vi "Sys B RX Host.vi"() -> ()   [LabVIEW 2019]
uses:
  SubVIs/mmWave HW Control/HW RX resources cluster.ctl
  <instrlib>/niMmWave/ni3610 and ni3630/controls/public/Board Information.ctl
  <instrlib>/niMmWave/ni3610 and ni3630/private/mm/Typedefs/PID.ctl
  <instrlib>/niMmWave/ni3610 and ni3630/controls/private/Board Hardware Revision.ctl
  SubVIs/mmWave HW Control/HW RX RF config cluster.ctl
  SubVIs/mmWave HW Control/HW Timing module config cluster.ctl
  SubVIs/mmWave HW Control/RX acquisition config.ctl
  SubVIs/Low-level/TypeDefs/TX trigger config.ctl
  FPGA/SubVIs/Utility/FPGA driver trigger source.ctl
  FPGA/SubVIs/Utility/FPGA driver trigger destination.ctl
  SubVIs/mmWave HW Control/Message and Data cluster.ctl
  SubVIs/mmWave HW Control/HW state enum.ctl
  <vilib>/Utility/error.llb/DialogType.ctl
  SubVIs/Low-level/TypeDefs/Hardware Configuration.ctl
  SubVIs/Low-level/TypeDefs/Direction.ctl
  SubVIs/Low-level/TypeDefs/Resources.ctl
  <vilib>/userdefined/High Color/nirio_resource_hc.ctl
  SubVIs/Low-level/TypeDefs/Front End Configuration.ctl
  SubVIs/Low-level/TypeDefs/Channel Configuration.ctl
  <instrlib>/niMmWave/ni3620/Config/v1/Host/Public/Typedefs/mmWave Port.ctl
  Intertarget communication/NS slave_class/NS slave.lvclass
  C:/Barkhausen mmWave radar/Development/LV/Barkhausen mmWave hardware control/Host/Intertarget communication/CR slave_class/CR slave.lvclass
  SubVIs/mmWave HW Control/mmWave HW Control.lvlib
  <instrlib>/niMmWave/ni3610 and ni3630/ni3610_and_ni3630_Driver_Lib.lvlib
  <instrlib>/niMmWave/ni3620/Config/v1/Host/niMmWave Config v1 Host.lvlib
  FPGA/SubVIs/Utility/FPGA Utility.lvlib
panel:
  out "SysA connected":bool
  in  "RX.Stop":bool
  out "Elements Remaining":u32
  out "Samples":u32
  in  "Stop Button":bool
  out "error out":T1
  out "Waveform plot":sgl[][](graph)
  in  "Tab Control":enum32{"HW setup", "Trigger setup"}(tab)
  in  "HW.RX resources":T2={"HW.IF"="IF_mod", "HW.ADC"="Rx_ADC", "HW.RX FPGA"="RX_FPGA"} caption="Reciever resources"
  in  "RX config":T3={"Gain"=0.0, "Frequency"=76000000000.0, "mmWave adapter"="mmWave0/0"} {"Frequency" format="%#_6fdb"; "Gain" format="%#_gdb"}
  in  "HW.init":bool
  in  "hw.conf trig":bool
  in  "HW.trig share config":T4={"mode"=enum."Import trig", "Timing module"="Dev1", "PXI line"="PXI_Trig1", "Module terminal"="PFI2"}
  in  "RX trigger options":T5={"delay"=136.0, "trig source"=enum."PXI_Trig", "PXI src"=1, "export"=enum."None", "PXI dest"=0}
  in  "Plot":bool=TRUE
  out "dt":dbl format="%#_6ps"
  in  "RX.read config":T8={"Samples"=16000}
  in  "RX.start":bool
  out "Rx information":T9={"product code"=30639, "hardware revision"=enum."Unknown", "serial number"=""} {"product code" items=["PXIe-3610 I/Q Generator"=30638, "PXIe-3630 I/Q Digitizer"=30639]}
  out "State":string
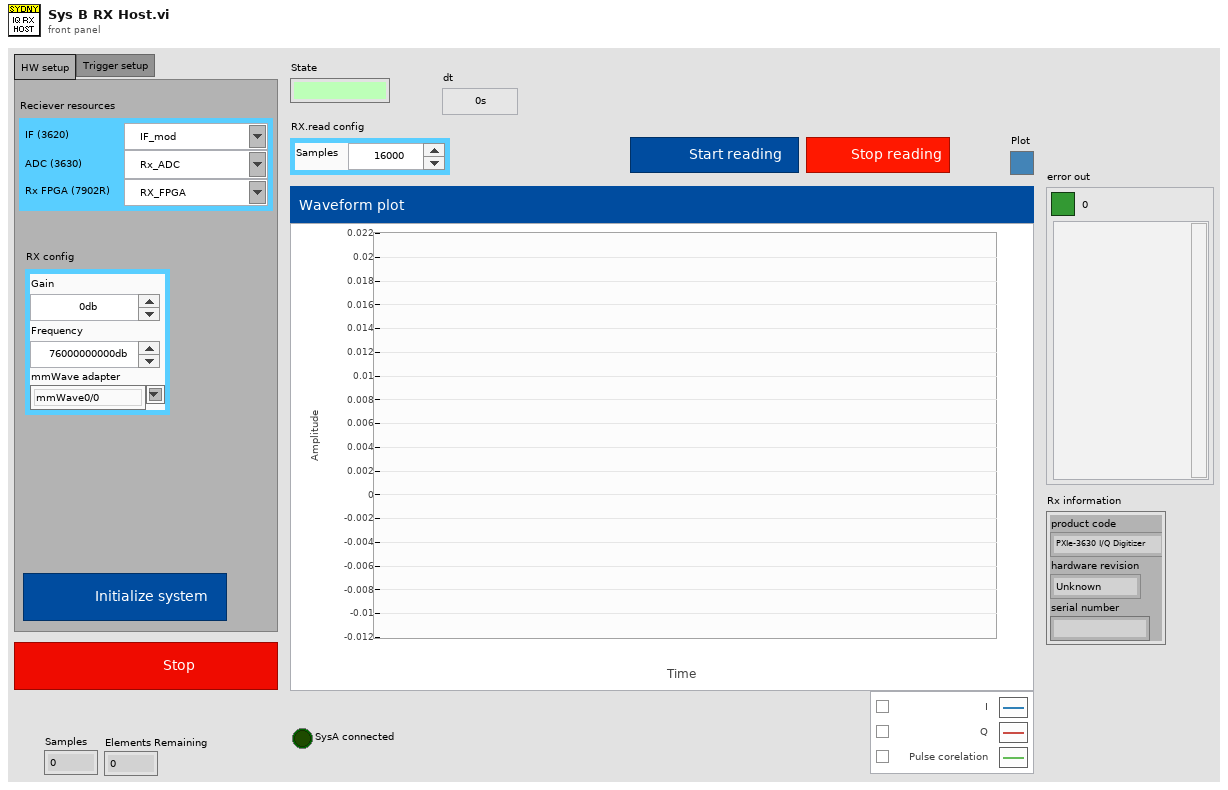
[diagram p1: front panel]
types:
  T1 = cluster{"Boolean Round":bool, "code":i32, "source":string}
  T2 = typedef "mmWave HW Control.lvlib/HW RX resources cluster.ctl" = cluster{"HW.IF":tag, "HW.ADC":refnum<visa-resource-name>, "HW.RX FPGA":tag}
  T3 = typedef "mmWave HW Control.lvlib/HW RX RF config cluster.ctl" = cluster{"Gain":dbl, "Frequency":dbl, "mmWave adapter":string}
  T4 = typedef "mmWave HW Control.lvlib/HW Timing module config cluster.ctl" = cluster{"mode":enum16{"None", "Export trig", "Import trig"}, "Timing module":tag, "PXI line":string, "Module terminal":string}
  T5 = typedef "TX trigger config.ctl" = cluster{"delay":dbl, "trig source":T6, "PXI src":i32, "export":T7, "PXI dest":i32}
  T6 = typedef "FPGA Utility.lvlib/FPGA driver trigger source.ctl" = enum16{"Use Tclk", "PXI_Trig", "Aurora RX trig"}
  T7 = typedef "FPGA Utility.lvlib/FPGA driver trigger destination.ctl" = enum16{"None", "Source trig", "Synced trig", "Delayed sync"}
  T8 = typedef "mmWave HW Control.lvlib/RX acquisition config.ctl" = cluster{"Samples":u32}
  T9 = typedef "Board Information.ctl" = cluster{"product code":T10, "hardware revision":T11, "serial number":string}
  T10 = typedef "ni3610_and_ni3630_Driver_Lib.lvlib/PID.ctl" = u16
  T11 = typedef "Board Hardware Revision.ctl" = enum16{"Unknown", "A", "B", "C", "D", "E", "F", "G", "H"}
  T12 = typedef "mmWave HW Control.lvlib/Message and Data cluster.ctl" = cluster{"message":string, "data":variant}
  T13 = typedef "mmWave HW Control.lvlib/HW state enum.ctl" = enum16{"idle", "configuration", "running", "exit"}
  T14 = typedef "Resources.ctl" = cluster{"7902R (Tx)":T15, "3610 (Tx)":refnum<visa-resource-name>, "3620 (IF)":T15, "3630 (RX)":refnum<visa-resource-name>, "7902R (Rx)":T15}
  T15 = typedef "nirio_resource_hc.ctl" = tag
  T16 = typedef "niMmWave Config v1 Host.lvlib/mmWave Port.ctl" = string
  T17 = typedef "Front End Configuration.ctl" = cluster{"port select":enum16{"IF Port", "Loopback", "Sync Port"}, "Rx hardware configuration":T18, "Tx hardware configuration":T18}
  T18 = typedef "Channel Configuration.ctl" = cluster{"gain (dB)":dbl, "frequency (Hz)":dbl, "mmWave adapter":string, "adapter active port":T16}
  T19 = typedef "DialogType.ctl" = u16
  T20 = typedef "Hardware Configuration.ctl" = cluster{"direction":T21, "baseband only":bool}
  T21 = typedef "Direction.ctl" = enum16{"Transceiver", "Receiver", "Transmitter"}
  T22 = typedef "Session.ctl" = cluster{"3620 session":refnum<queue>, "tx baseband session":T23, "rx baseband session":T31, "tx gain (dB)":dbl, "rx gain (dB)":dbl, "hardware configuration":T20, "gain ranging":T32[], "pxi trigger bus information":T33}
  T23 = typedef "Tx Baseband Session.ctl" = cluster{"3610 session":T24, "7902 reference":T30}
  T24 = typedef "ni3610_and_ni3630_Driver_Lib.lvlib/Main Settings.ctl" = cluster{"VISA resource name":refnum<visa-resource-name>, "Address Space":T25, "window_offset":u32, "register_addresses":T26, "required_MM_fpga_version":cluster{"signature":u32, "hardware":u32, "current revision":u32, "oldest revision":u32}, "CPLD Oldest Compat Version ":cluster{"hardware":u32, "CPLD firmware":u32}, "MM_FPGA_image_location":string, "is_init":bool, "card_type":T27, "DacLmkConfigFileName":string, "AdcLmkConfigFileName":string, "AdcConfigFileName":string, "DacConfigFileName_RevA":string, "DacConfigFileName_RevB":string, "Mulde hardware revision":u8, "bypass DAC PLL\n":bool, "IQ Card Revision":T28, "board capability":T29}
  T25 = typedef "VISA Register Access Address Space.ctl" = u16
  T26 = typedef "ni3610_and_ni3630_Driver_Lib.lvlib/Register Adresses.ctl" = cluster{"MM based Registers":cluster{"Revision":u32, "OldestCompatRev":u32, "signature":u32, "scratch":u32, "LedControl":u32, "BoardHwRev":u32, "BoardControl":u32, "ThermalStatus":u32, "BasebandStatus":u32, "BasebandControl":u32, "BasebandAuxSetup":u32, "BasebandAuxStatus":u32, "LmkSyncOutSetup":u32, " AdcSyncOutSetup":u32, " InjSyncOutSetup":u32, " PxiTrig0OutSetup":u32, " PxiTrig1OutSetup":u32, " PxiTrig2OutSetup":u32, " PxiTrig3OutSetup":u32, " PxiTrig4OutSetup":u32, " PxiTrig5OutSetup":u32, " PxiTrig6OutSetup":u32, " PxiTrig7OutSetup":u32}, "CPLD based Registers":cluster{"SlaveSignature":u32, "SlaveRevision":u32, "SlaveOldestCompatRev":u32, "SlaveScratch":u32, "SlaveSetup":u32, "SlaveStatus":u32, "IDacReg_offset":u32, "LMKRegGrp0_offset":u32, "QDacReg_offset":u32, "BrdTempSensorVal":u32, "TempSensorPowerDown":u32, "GPIOReg_offset":u32, "IAdcReg_offset":u32, "QAdcReg_offset":u32, "LMKRegGrp1_offset":u32, "QadcTempSensorVal":u32, "IadcTempSensorVal":u32, "RevisionReg":u32, "VcxoReg":u32, "CpldStatusReg":u32, "PowerReg":u32, "VBiasEnReg":u32, "ExtRefOeReg":u32, "QdacCtrlReg":u32, "QdacStatusReg":u32, "IdacCtrlReg":u32, "IdacStatusReg":u32, "QdacJtagIn":u32, "QdacJtagOut":u32, "IdacJtagIn":u32, "IdacJtagOut":u32, "IqDcSetupReg":u32, "QadcStatusReg":u32, "IadcStatusReg":u32, "BrdSetupReg":u32, "IqDcRevisionReg":u32, "PllStatusReg":u32, "EndpointScratchReg":u32, "AdcSyncCfgReg":u32, "IqCardOpampReg":u32}, "CPLD Register Offset":u32, "MM  Register Offset":u32, " PxiTrig0OutSetup":u32}
  T27 = typedef "ni3610_and_ni3630_Driver_Lib.lvlib/Base Card Type.ctl" = enum16{"unspecified", "ADC", "DAC"}
  T28 = typedef "ni3610_and_ni3630_Driver_Lib.lvlib/IQ Card Revision.ctl" = enum16{"RevA", "RevB", "RevC", "RevD"}
  T29 = typedef "ni3610_and_ni3630_Driver_Lib.lvlib/Board Capability.ctl" = cluster{"baseband sync":enum16{"no baseband sync", "baseband sync"}}
  T30 = typedef "Blank FPGA Reference.ctl" = refnum<k20>
  T31 = typedef "Rx Baseband Session.ctl" = cluster{"3630 session":T24, "7902 reference":T30}
  T32 = typedef "Gain Ranging.ctl" = cluster{"gain ranging active scope":string, "gain ranging stream session":refnum<k20>}
  T33 = typedef "PXI Trigger Bus Info.ctl" = cluster{"chassis resource name":refnum<visa-resource-name>, "7902R (TX)":i16, "3610 (TX)":i16, "3620 (IF)":i16, "3630 (RX)":i16, "7902R (RX)":i16}
  T34 = typedef "Constants.ctl" = cluster{"data clock rate (Hz)":dbl, "sample rate (Hz)":dbl, "sample rate selector string":string, "default tx bitfile path":path, "default rx bitfile path":path, "default proc bitfile path":path}
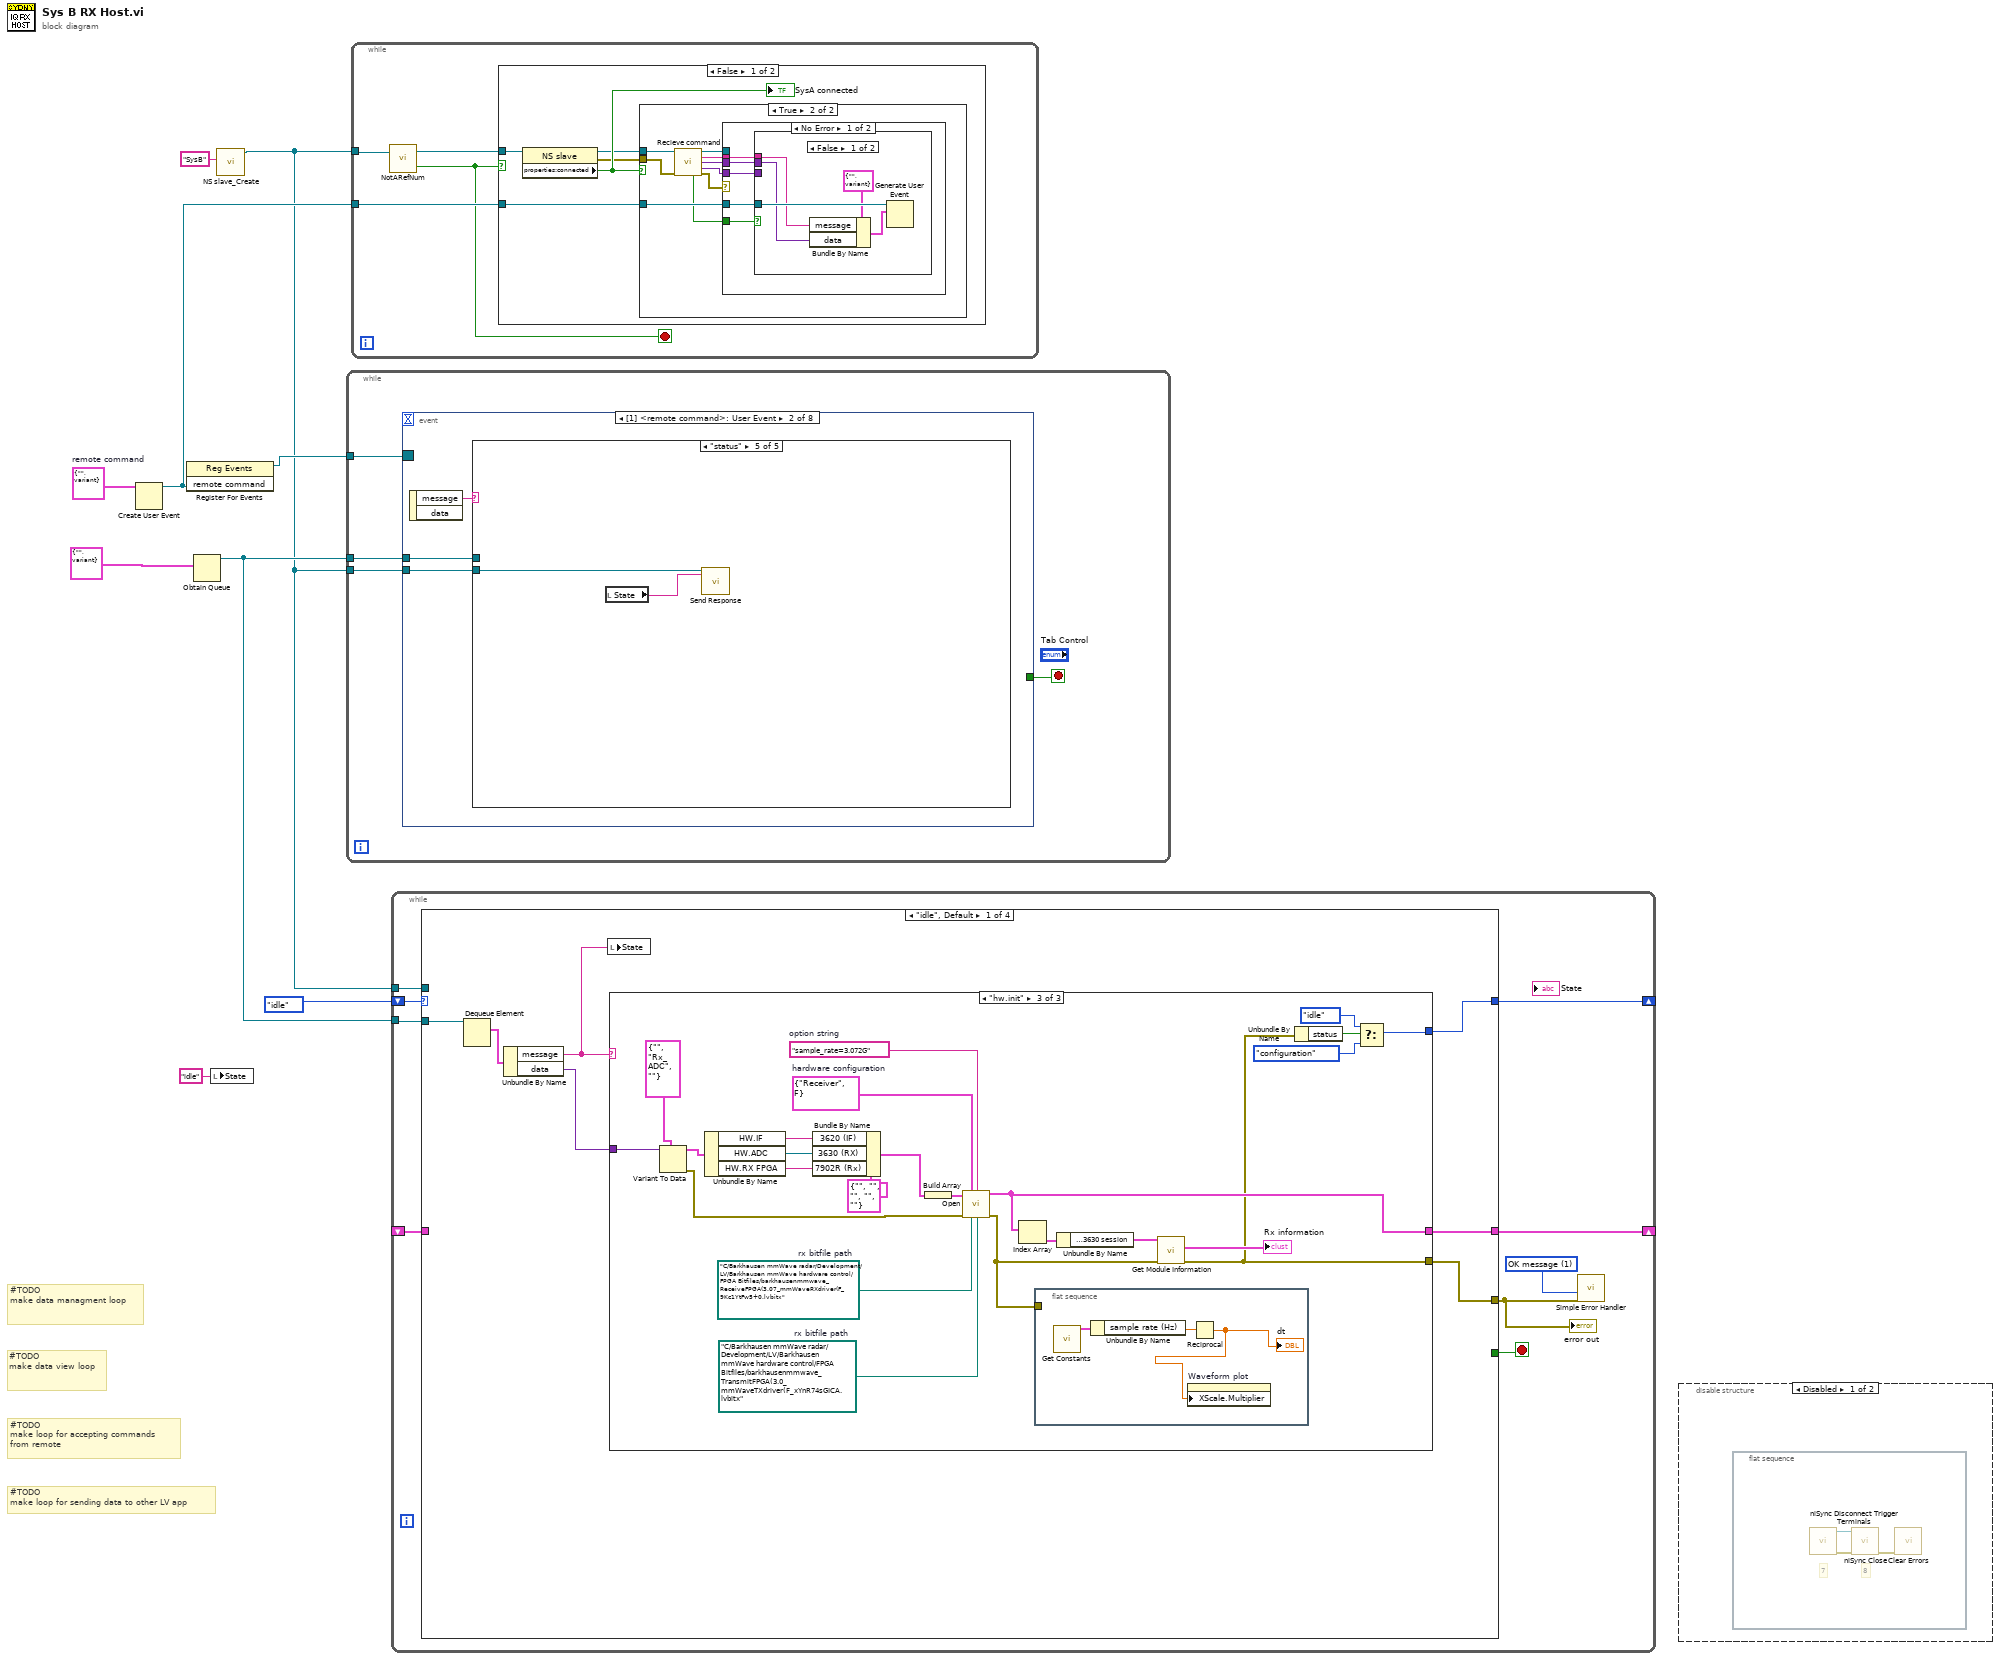
[diagram p0: block diagram]
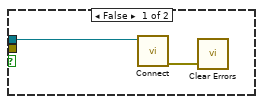
[diagram p2: hidden frame]
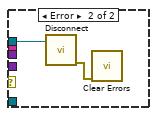
[diagram p4: hidden frame]
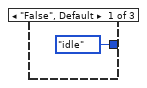
[diagram p7: hidden frame]
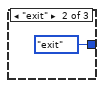
[diagram p8: hidden frame]
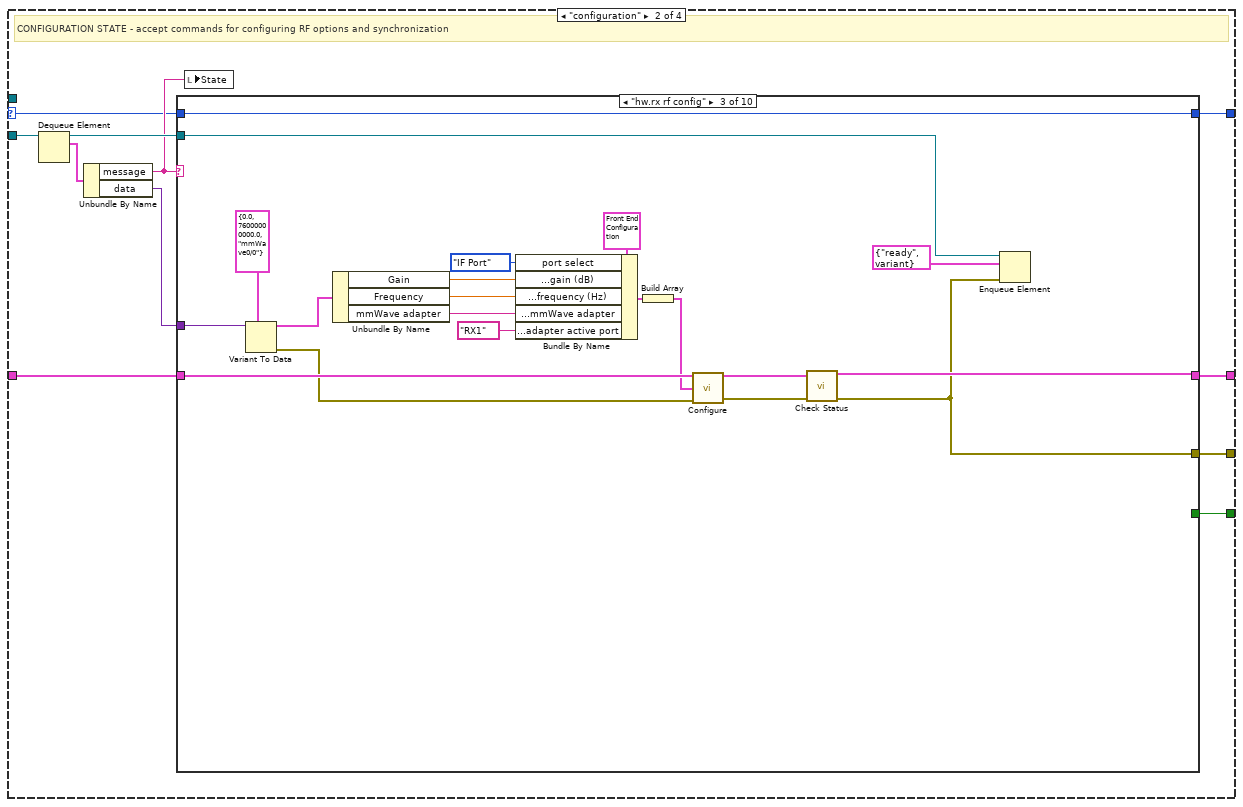
[diagram p9: hidden frame]
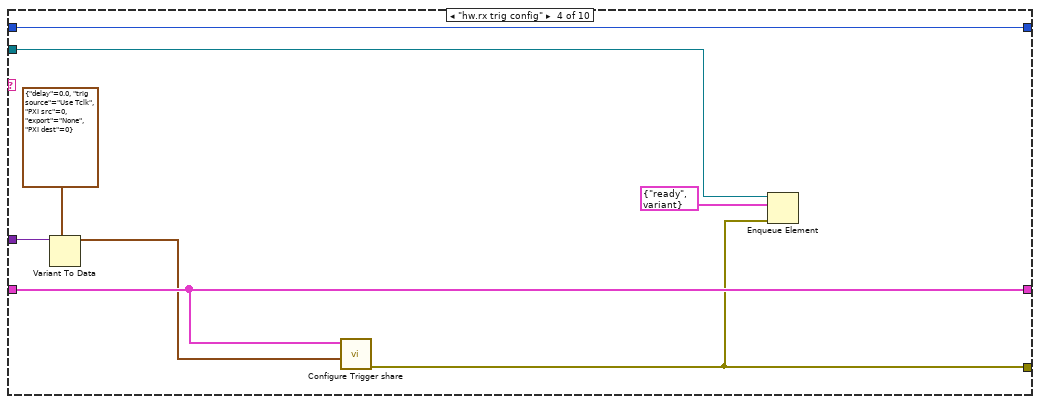
[diagram p12: hidden frame]
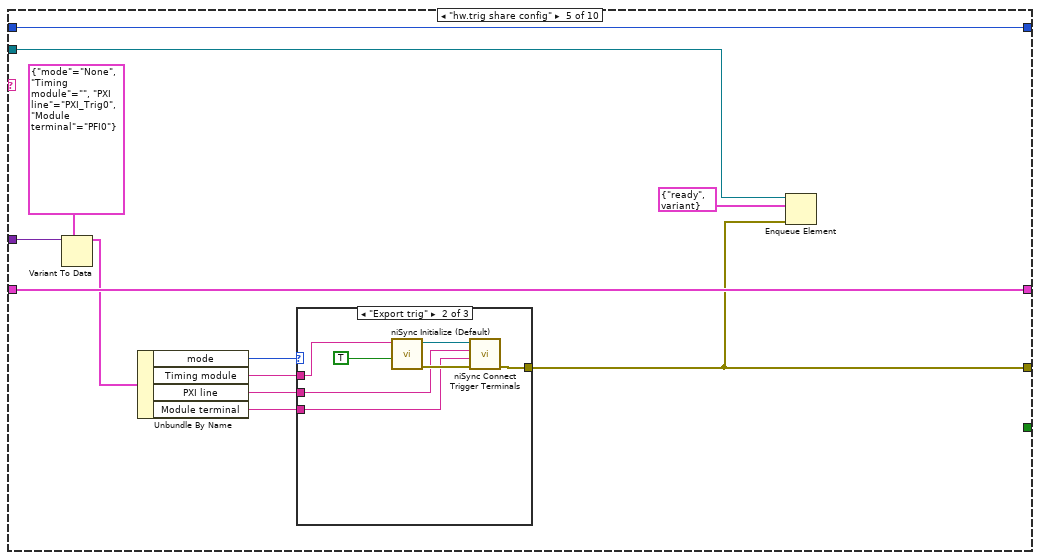
[diagram p13: hidden frame]
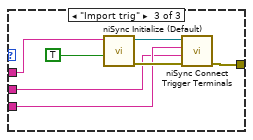
[diagram p15: hidden frame]
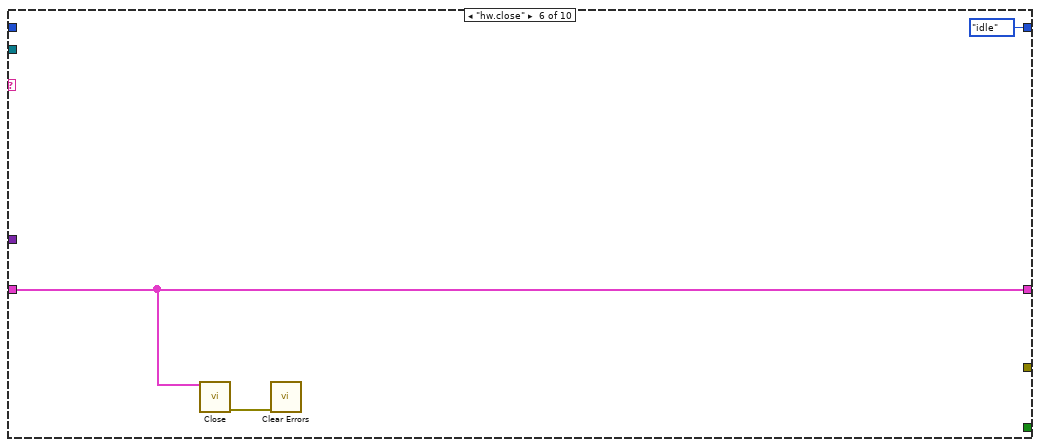
[diagram p16: hidden frame]
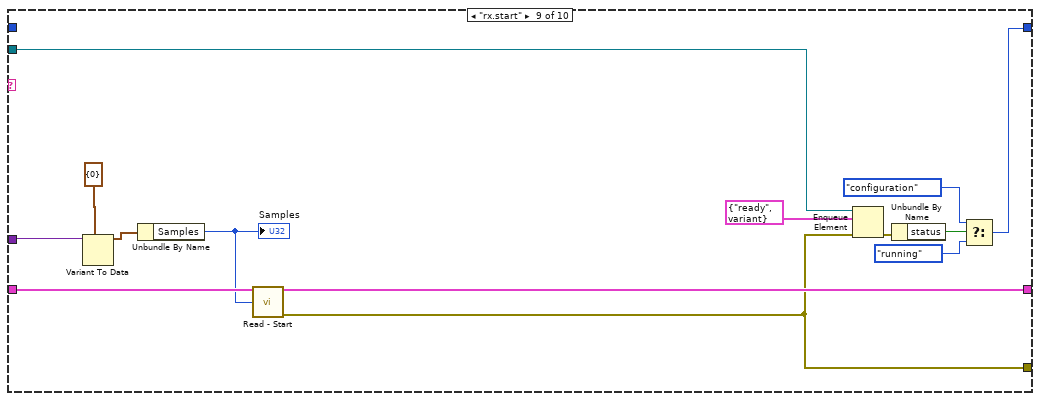
[diagram p19: hidden frame]
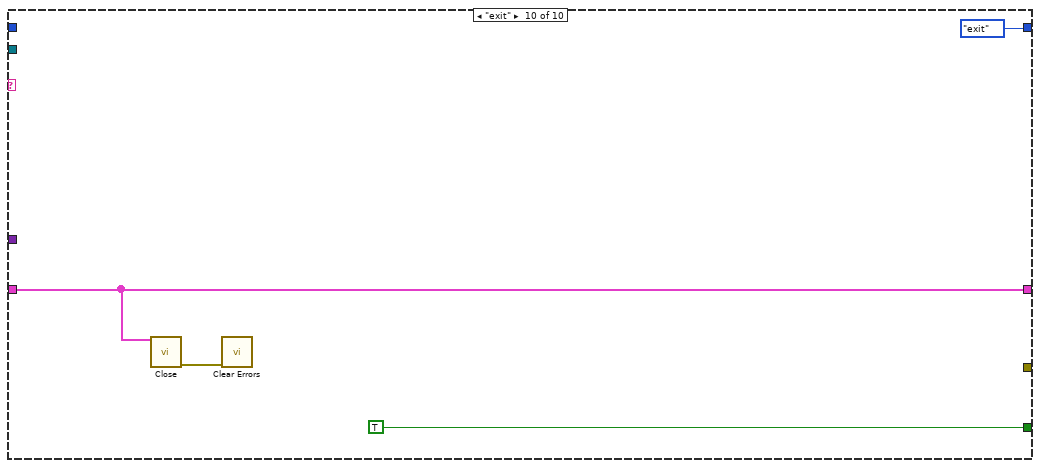
[diagram p20: hidden frame]
diagram:
  w4 = T12 {"message"="", "data"=variant}  # remote command
  # "#TODO\nmake loop for sending data to other LV app"
  # "#TODO\nmake loop for accepting commands\nfrom remote"
  # "#TODO\nmake data view loop"
  # "#TODO\nmake data managment loop"
  n1 = Create User Event(user event datatype=w4) -> (user event=w3:refnum<user-event>)  [unwired: 1 in, 1 out]
  n2 = register-events(w3) -> (reference out=w2:refnum<event-registration>)  [unwired: 2 in, 1 out]
  n3 = Obtain Queue(element data type=T12 {"message"="", "data"=variant} ("Message data cluster")) -> (queue out=w9:refnum<queue>)  [unwired: 4 in, 2 out]
  n4 = local write "State"("idle" ("State")) -> ()
  n5 = call "NS slave_Create.vi"("ID"="SysB") -> ("reference out"=w1:refnum<class "NS slave.lvclass">)  [unwired: 9 in, 1 out]
  n6 = while {
    tunnel: w9 -> [w12]
    tunnel: w2 -> [w11]
    tunnel: w1 -> [w10]
    stop <- w13 stop-if-true
    n7 = event shown="[1] <remote command>: User Event" {
      selector: w11 -> [_ _ _ _ _ _ _ _]
      dyn-events: _ -> [_ _ _ _ _ _ _ _]
      timeout: _ -> [_ _ _ _ _ _ _ _]
      tunnel: [_ _ TRUE _ _ _ _ _] -> w13
      tunnel: w12 -> [_ w15 w56 w60 w89 w91 w98 w104]
      tunnel: w10 -> [_ w14 w54 _ _ _ _ _]
      event Timeout {
        n8 = event-data() -> ()  [unwired: 1 in, 3 out]
      }
      event User Event {
        n9 = event-data() -> ("message"=w16:string)  [unwired: 1 in, 1 out]
        n10 = case shown="\"status\"" w16 {
          tunnel: w15 -> [_ w18 w41 w49 _]
          tunnel: w14 -> [_ _ _ _ w52]
          frame "False", Default {
          }
          frame "hw.reinit" {
            n11 = local read "HW.RX resources"() -> (w25:T2)
            n12 = local read "RX config"() -> (w38:T3)
            n13 = local read "RX trigger options"() -> (w31:T5)
            n14 = local read "HW.trig share config"() -> (w32:T4)
            n15 = Enqueue Element(queue=w18, element=T12 {"message"="hw.close", "data"=variant}) -> (queue out=w17:refnum<queue>)  [unwired: 2 in, 2 out]
            n16 = Bundle By Name(cluster=T12 {"message"="hw.init", "data"=variant} ("element"), "data"=w25) -> (w40:T12)
            n17 = Bundle By Name(cluster=T12 {"message"="hw.rx rf config", "data"=variant} ("element"), "data"=w38) -> (w36:T12)
            n18 = Bundle By Name(cluster=T12 {"message"="hw.rx trig config", "data"=variant} ("element"), "data"=w31) -> (w35:T12)
            n19 = Bundle By Name(cluster=T12 {"message"="hw.trig share config", "data"=variant} ("element"), "data"=w32) -> (w33:T12)
            n20 = Enqueue Element(queue=w17, element=w40) -> (queue out=w39:refnum<queue>, error out=w29:errorcluster)  [unwired: 2 in, 1 out]
            n21 = Enqueue Element(queue=w39, element=w36, error in (no error)=w29) -> (queue out=w37:refnum<queue>, error out=w28:errorcluster)  [unwired: 1 in, 1 out]
            n22 = Enqueue Element(queue=w37, element=w35, error in (no error)=w28) -> (queue out=w34:refnum<queue>, error out=w27:errorcluster)  [unwired: 1 in, 1 out]
            n23 = Enqueue Element(queue=w34, element=w33, error in (no error)=w27) -> (queue out=w30:refnum<queue>, error out=w26:errorcluster)  [unwired: 1 in, 1 out]
            n24 = Enqueue Element(queue=w30, element=T12 {"message"="ready", "data"=variant}, error in (no error)=w26) -> ()  [unwired: 1 in, 3 out]
          }
          frame "rx.start" {
            n25 = local read "RX trigger options"() -> (w45:T5)
            n26 = local read "RX.read config"() -> (w44:T8)
            n27 = Bundle By Name(cluster=T12 {"message"="rx.start", "data"=variant} ("element"), "data"=w44) -> (w48:T12)
            n28 = Bundle By Name(cluster=T12 {"message"="hw.rx trig config", "data"=variant} ("element"), "data"=w45) -> (w47:T12)
            n29 = Enqueue Element(queue=w41, element=w47) -> (queue out=w46:refnum<queue>)  [unwired: 2 in, 2 out]
            n30 = Enqueue Element(queue=w46, element=w48) -> ()  [unwired: 2 in, 3 out]
          }
          frame "rx.stop" {
            n31 = Enqueue Element(queue=w49, element=T12 {"message"="rx.stop read", "data"=variant}) -> ()  [unwired: 2 in, 3 out]
          }
          frame "status" {
            n32 = local read "State"() -> (w51:string)
            n33 = call-dynamic "Send Response.vi"("reference in"=w52, "response"=w51) -> ()  [unwired: 16 in, 2 out]
          }
        }
      }
      event "Stop Button": Value Change {
        n34 = event-data() -> ()  [unwired: 1 in, 6 out]
        n35 = call-dynamic "Destroy.vi"("reference in"=w54) -> ("error out"=w53:errorcluster)  [unwired: 17 in, 1 out]
        n36 = Enqueue Element(queue=w56, element=T12 {"message"="exit", "data"=variant}) -> ()  [unwired: 2 in, 3 out]
        n37 = call <vilib>:"Clear Errors.vi"("error in (no error)"=w53) -> ()  [unwired: 5 in, 2 out]
      }
      event "HW.init": Value Change {
        n38 = event-data() -> ()  [unwired: 1 in, 3 out]
        n39 = local read "HW.RX resources"() -> (w62:T2)
        n40 = local read "RX config"() -> (w78:T3)
        n41 = local read "RX trigger options"() -> (w69:T5)
        n42 = local read "HW.trig share config"() -> (w70:T4)
        n43 = Enqueue Element(queue=w60, element=T12 {"message"="hw.close", "data"=variant}) -> (queue out=w59:refnum<queue>, error out=w58:errorcluster)  [unwired: 2 in, 1 out]
        n44 = Bundle By Name(cluster=T12 {"message"="hw.init", "data"=variant} ("element"), "data"=w62) -> (w81:T12)
        n45 = Bundle By Name(cluster=T12 {"message"="hw.rx rf config", "data"=variant} ("element"), "data"=w78) -> (w76:T12)
        n46 = Bundle By Name(cluster=T12 {"message"="hw.rx trig config", "data"=variant} ("element"), "data"=w69) -> (w74:T12)
        n47 = Bundle By Name(cluster=T12 {"message"="hw.trig share config", "data"=variant} ("element"), "data"=w70) -> (w71:T12)
        n48 = Enqueue Element(queue=w59, element=w81, error in (no error)=w58) -> (queue out=w80:refnum<queue>, error out=w66:errorcluster)  [unwired: 1 in, 1 out]
        n49 = Enqueue Element(queue=w80, element=w76, error in (no error)=w66) -> (queue out=w77:refnum<queue>, error out=w65:errorcluster)  [unwired: 1 in, 1 out]
        n50 = Enqueue Element(queue=w77, element=w74, error in (no error)=w65) -> (queue out=w73:refnum<queue>, error out=w64:errorcluster)  [unwired: 1 in, 1 out]
        n51 = Enqueue Element(queue=w73, element=w71, error in (no error)=w64) -> (queue out=w68:refnum<queue>, error out=w63:errorcluster)  [unwired: 1 in, 1 out]
        n52 = Enqueue Element(queue=w68, element=T12 {"message"="ready", "data"=variant}, error in (no error)=w63) -> ()  [unwired: 1 in, 3 out]
      }
      event "hw.conf trig": Value Change {
        n53 = event-data() -> ()  [unwired: 1 in, 6 out]
        n54 = Bundle By Name(cluster=T12 {"message"="hw.rx trig config", "data"=variant} ("element"), "data"="RX trigger options") -> (w86:T12)
        n55 = Bundle By Name(cluster=T12 {"message"="hw.trig share config", "data"=variant} ("element"), "data"="HW.trig share config") -> (w85:T12)
        n56 = Enqueue Element(queue=w89, element=w86) -> (queue out=w90:refnum<queue>)  [unwired: 2 in, 2 out]
        n57 = Enqueue Element(queue=w90, element=w85) -> ()  [unwired: 2 in, 3 out]
      }
      event Value Change {
        n58 = event-data() -> ()  [unwired: 1 in, 6 out]
        n59 = Bundle By Name(cluster=T12 {"message"="hw.rx rf config", "data"=variant} ("element"), "data"="RX config") -> (w94:T12)
        n60 = Enqueue Element(queue=w91, element=w94) -> ()  [unwired: 2 in, 3 out]
      }
      event "RX.start": Value Change {
        n61 = event-data() -> ()  [unwired: 1 in, 2 out]
        n62 = local read "RX trigger options"() -> (w96:T5)
        n63 = local read "RX.read config"() -> (w95:T8)
        n64 = Bundle By Name(cluster=T12 {"message"="rx.start", "data"=variant} ("element"), "data"=w95) -> (w101:T12)
        n65 = Bundle By Name(cluster=T12 {"message"="hw.rx trig config", "data"=variant} ("element"), "data"=w96) -> (w99:T12)
        n66 = Enqueue Element(queue=w98, element=w99) -> (queue out=w97:refnum<queue>)  [unwired: 2 in, 2 out]
        n67 = Enqueue Element(queue=w97, element=w101) -> ()  [unwired: 2 in, 3 out]
      }
      event "RX.Stop": Value Change {
        n68 = event-data() -> ()  [unwired: 1 in, 2 out]
        n69 = Enqueue Element(queue=w104, element=T12 {"message"="rx.stop read", "data"=variant}) -> ()  [unwired: 2 in, 3 out]
      }
    }
  }
  n70 = while {
    tunnel: w1 -> [w108]
    tunnel: w3 -> [w106]
    stop <- w105 stop-if-true
    n71 = call-dynamic "NotARefNum.vi"("reference in"=w108) -> ("not a refnum?"=w105:bool, "reference out"=w107:refnum<class "NS slave.lvclass">)  [unwired: 1 in]
    n72 = case shown="False" w105 {
      tunnel: w107 -> [w113 _]
      tunnel: w106 -> [w110 _]
      frame False {
        n73 = property class="NS slave"(reference=w113) -> (reference out=w111:refnum<class "NS slave.lvclass">, error out=w109:errorcluster, "properties:connected"=w112:bool)  [unwired: 1 in]
        "SysA connected" <- w112
        n74 = case shown="True" w112 {
          tunnel: w111 -> [w115 w124]
          tunnel: w110 -> [_ w123]
          tunnel: w109 -> [_ w119]
          frame False {
            n75 = call-dynamic "Connect.vi"("reference in"=w115) -> ("error out"=w114:errorcluster)  [unwired: 9 in, 1 out]
            n76 = call <vilib>:"Clear Errors.vi"("error in (no error)"=w114) -> ()  [unwired: 5 in, 2 out]
          }
          frame True {
            n77 = call-dynamic "Recieve command.vi"("reference in"=w124, "error in (no error)"=w119) -> ("reference out"=w118:refnum<class "NS slave.lvclass">, "message"=w122:string, "parameters"=w121:variant, "data"=w120:variant, "timed out?"=w116:bool, "error out"=w117:errorcluster)  [unwired: 8 in]
            n78 = case shown="No Error" w117 {
              tunnel: w123 -> [w129 _]
              tunnel: w122 -> [w128 _]
              tunnel: w121 -> [w127 _]
              tunnel: w120 -> [w126 _]
              tunnel: w118 -> [_ w135]
              tunnel: w116 -> [w125 _]
              frame No Error {
                n79 = case shown="False" w125 {
                  tunnel: w129 -> [w134 _]
                  tunnel: w128 -> [w132 _]
                  tunnel: w127 -> [w131 _]
                  tunnel: w126 -> [_ _]
                  frame False {
                    n80 = Bundle By Name(cluster=T12 {"message"="", "data"=variant}, "message"=w132, "data"=w131) -> (w130:T12)
                    n81 = Generate User Event(user event=w134, event data cluster=w130) -> ()  [unwired: 2 in, 2 out]
                  }
                  frame True {
                  }
                }
              }
              frame Error {
                n82 = call-dynamic "Disconnect.vi"("reference in"=w135) -> ("error out"=w136:errorcluster)  [unwired: 9 in, 1 out]
                n83 = call <vilib>:"Clear Errors.vi"("error in (no error)"=w136) -> ()  [unwired: 5 in, 2 out]
              }
            }
          }
        }
      }
      frame True {
      }
    }
  }
  n84 = while {
    tunnel: w9 -> [w141]
    shift-right: [w144] -> _
    shift-left: _ -> [w143]
    shift-right: [w138] -> _
    shift-left: HW_state_enum."idle" ("hw state") -> [w139]
    tunnel: w1 -> [w137]
    stop <- w145 stop-if-true
    w140 = T19 1 items=["no dialog", "OK message", "continue or stop message", "OK message + warnings", "continue/stop + warnings"] ("type of dialog (OK msg:1)")
    n85 = case shown="\"idle\", Default" w139 {
      selector: w139 -> [_ w183 w285 w328]
      tunnel: [_ w191 w276 TRUE] -> w145
      tunnel: [w148 w189 w280 w327] -> w144
      tunnel: w143 -> [_ w188 w281 w327]
      tunnel: [w146 w187 w279 _] -> w142
      tunnel: w141 -> [w151 w186 w287 _]
      tunnel: [w147 w182 w282 w328] -> w138
      tunnel: w137 -> [_ _ w277 _]
      frame "idle", Default {
        n86 = Dequeue Element(queue=w151) -> (element=w152:T12)  [unwired: 2 in, 3 out]
        n87 = Unbundle By Name(w152) -> ("message"=w150:string, "data"=w149:variant)
        n88 = local write "State"(w150) -> ()
        n89 = case shown="\"hw.init\"" w150 {
          tunnel: w149 -> [_ _ w161]
          tunnel: [_ _ w160] -> w148
          tunnel: [HW_state_enum."idle" ("hw state") HW_state_enum."exit" ("hw state") w156] -> w147
          tunnel: [_ _ w155] -> w146
          frame "False", Default {
          }
          frame "exit" {
          }
          frame "hw.init" {
            w165 = "sample_rate=3.072G"  # option string
            w164 = path "C:/Barkhausen mmWave radar/Development/LV/Barkhausen mmWave hardware control/FPGA Bitfiles/barkhausenmmwave_ReceiveFPGA(3.07_mmWaveRXdriver(F_9Kc1YtFw5+0.lvbitx"  # rx bitfile path
            w163 = path "C:/Barkhausen mmWave radar/Development/LV/Barkhausen mmWave hardware control/FPGA Bitfiles/barkhausenmmwave_TransmitFPGA(3.0_mmWaveTXdriver(F_xYnR74sGICA.lvbitx"  # rx bitfile path
            w177 = T20 {"direction"=enum."Receiver", "baseband only"=FALSE}  # hardware configuration
            n90 = Variant To Data(type=T2 {"HW.IF"="", "HW.ADC"="Rx_ADC", "HW.RX FPGA"=""} ("HW.RX devices"), Variant=w161) -> (data=w178:T2, error out=w168:errorcluster)  [unwired: 1 in]
            n91 = Unbundle By Name(w178) -> ("HW.IF"=w174:tag, "HW.ADC"=w173:refnum<visa-resource-name>, "HW.RX FPGA"=w172:tag)
            n92 = Bundle By Name(cluster=T14 {"7902R (Tx)"="", "3610 (Tx)"="", "3620 (IF)"="", "3630 (RX)"="", "7902R (Rx)"=""} ("resources"), "3620 (IF)"=w174, "3630 (RX)"=w173, "7902R (Rx)"=w172) -> (w176:T14)
            n93 = Build Array(w176) -> (w175:T14[])
            n94 = call "Open.vi"("resources"=w175, "hardware configuration"=w177, "option string"=w165, "error in"=w168, "rx bitfile path"=w164, "tx bitfile path"=w163) -> ("session out"=w160:T22[], "error out"=w167:errorcluster)  [unwired: 7 in, 1 out]
            n95 = Index Array(array=w160) -> (element=w171:T22)  [unwired: 1 in]
            n96 = flat-sequence {
              tunnel: w167 -> [_]
              frame #0 {
                n97 = call "Get Constants.vi"() -> ("constants"=w181:T34)  [unwired: 15 in]
                n98 = Unbundle By Name(w181) -> ("sample rate (Hz)"=w180:dbl)
                n99 = Reciprocal(x=w180) -> (1/x=w179:dbl)
                "dt" <- w179
                n100 = property on="Waveform plot" class="WFGraph (strict)"("XScale.Multiplier"=w179) -> ()  [unwired: 2 in, 2 out]
              }
            }
            n101 = Unbundle By Name(w171) -> ("rx baseband session.3630 session"=w170:T24)
            n102 = call <instrlib>:"Get Module Information.vi"("error in (no error)"=w167, "Board Settings in"=w170) -> ("error out"=w155:errorcluster, "board information"=→"Rx information":T9)  [unwired: 7 in, 1 out]
            n103 = Unbundle By Name(w155) -> ("status"=w159:bool)
            n104 = Select(t=HW_state_enum."idle" ("hw state"), s=w159, f=HW_state_enum."configuration" ("hw state")) -> (s? t:f=w156:T13)
          }
        }
      }
      frame "configuration" {
        # "CONFIGURATION STATE - accept commands for configuring RF options and synchronization"
        n105 = Dequeue Element(queue=w186) -> (queue out=w185:refnum<queue>, element=w192:T12)  [unwired: 2 in, 2 out]
        n106 = Unbundle By Name(w192) -> ("message"=w184:string, "data"=w190:variant)
        n107 = case shown="\"hw.rx rf config\"" w184 {
          tunnel: [_ _ _ _ _ _ _ _ _ TRUE] -> w191
          tunnel: w190 -> [_ _ w216 w224 w235 _ _ _ w271 _]
          tunnel: [w194 w196 w203 w222 w236 w251 w255 w257 w259 w274] -> w189
          tunnel: w188 -> [w194 w196 w214 w222 w236 w251 w255 w257 w261 w274]
          tunnel: [_ _ w199 w218 w226 _ _ _ w258 _] -> w187
          tunnel: w185 -> [_ _ w200 w219 w227 _ _ _ w268 _]
          tunnel: w183 -> [w193 w195 w198 w217 w225 _ w254 w256 _ _]
          tunnel: [w193 w195 w198 w217 w225 HW_state_enum."idle" ("hw state") w254 w256 w262 HW_state_enum."exit" ("hw state")] -> w182
          frame Default {
          }
          frame "----HARDWARE CONFIG----" {
          }
          frame "hw.rx rf config" {
            n108 = Variant To Data(type=T3 {"Gain"=0.0, "Frequency"=76000000000.0, "mmWave adapter"="mmWave0/0"} ("RX config"), Variant=w216) -> (data=w213:T3, error out=w202:errorcluster)  [unwired: 1 in]
            n109 = Unbundle By Name(w213) -> ("Gain"=w206:dbl, "Frequency"=w207:dbl, "mmWave adapter"=w208:string)
            n110 = Bundle By Name(cluster=T17 {"port select"=enum."Loopback", "Rx hardware configuration"={"gain (dB)"=15.0, "frequency (Hz)"=12000000000.0, "mmWave adapter"="None", "adapter active port"=""}, "Tx hardware configuration"={"gain (dB)"=-15.0, "frequency (Hz)"=12000000000.0, "mmWave adapter"="None", "adapter active port"=""}} ("device configuration [channel]"), "port select"=enum16{"IF Port", "Loopback", "Sync Port"}."IF Port", "Rx hardware configuration.gain (dB)"=w206, "Rx hardware configuration.frequency (Hz)"=w207, "Rx hardware configuration.mmWave adapter"=w208, "Rx hardware configuration.adapter active port"=T16 "RX1") -> (w210:T17)
            n111 = Build Array(w210) -> (w209:T17[])
            n112 = call "Configure.vi"("session in"=w214, "device configuration [channel]"=w209, "error in"=w202) -> ("session out"=w205:T22[], "error out"=w204:errorcluster)  [unwired: 10 in, 1 out]
            n113 = call "Check Status.vi"("session in"=w205, "error in"=w204) -> ("session out"=w203:T22[], "error out"=w199:errorcluster)  [unwired: 9 in, 3 out]
            n114 = Enqueue Element(queue=w200, element=T12 {"message"="ready", "data"=variant}, error in (no error)=w199) -> ()  [unwired: 1 in, 3 out]
          }
          frame "hw.rx trig config" {
            n115 = Variant To Data(type=T5 {"delay"=0.0, "trig source"=enum."Use Tclk", "PXI src"=0, "export"=enum."None", "PXI dest"=0} ("RX trigger options"), Variant=w224) -> (data=w221:T5)  [unwired: 1 in, 1 out]
            n116 = call "Configure Trigger share.vi"("RX trigger options"=w221, "session in"=w222) -> ("error out"=w218:errorcluster)  [unwired: 6 in, 3 out]
            n117 = Enqueue Element(queue=w219, element=T12 {"message"="ready", "data"=variant}, error in (no error)=w218) -> ()  [unwired: 1 in, 3 out]
          }
          frame "hw.trig share config" {
            n118 = Variant To Data(type=T4 {"mode"=enum."None", "Timing module"="", "PXI line"="PXI_Trig0", "Module terminal"="PFI0"} ("HW.trig share config"), Variant=w235) -> (data=w233:T4)  [unwired: 1 in, 1 out]
            n119 = Unbundle By Name(w233) -> ("mode"=w232:enum16{"None", "Export trig", "Import trig"}, "Timing module"=w231:tag, "PXI line"=w230:string, "Module terminal"=w229:string)
            n120 = case shown="\"Export trig\"" w232 {
              tunnel: w231 -> [_ w240 w247]
              tunnel: [_ w239 w246] -> w226
              tunnel: w230 -> [_ w238 w244]
              tunnel: w229 -> [_ w237 w245]
              frame "None", Default {
              }
              frame "Export trig" {
                n121 = call <instrlib>:"niSync Initialize (Default).vi"("reset device (F)"=TRUE ("reset device (False)"), "resource name"=w240) -> ("error out"=w243:errorcluster, "instrument handle out"=w242:refnum<k15>)  [unwired: 8 in]
                n122 = call <instrlib>:"niSync Connect Trigger Terminals.vi"("error in (no error)"=w243, "destination terminal"=w237, "source terminal"=w238, "instrument handle"=w242) -> ("error out"=w239:errorcluster)  [unwired: 6 in, 1 out]
              }
              frame "Import trig" {
                n123 = call <instrlib>:"niSync Initialize (Default).vi"("reset device (F)"=TRUE ("reset device (False)"), "resource name"=w247) -> ("error out"=w250:errorcluster, "instrument handle out"=w249:refnum<k15>)  [unwired: 8 in]
                n124 = call <instrlib>:"niSync Connect Trigger Terminals.vi"("error in (no error)"=w250, "destination terminal"=w244, "source terminal"=w245, "instrument handle"=w249) -> ("error out"=w246:errorcluster)  [unwired: 6 in, 1 out]
              }
            }
            n125 = Enqueue Element(queue=w227, element=T12 {"message"="ready", "data"=variant}, error in (no error)=w226) -> ()  [unwired: 1 in, 3 out]
          }
          frame "hw.close" {
            n126 = call "Close.vi"("session"=w251) -> ("error out"=w252:errorcluster)  [unwired: 14 in]
            n127 = call <vilib>:"Clear Errors.vi"("error in (no error)"=w252) -> ()  [unwired: 5 in, 2 out]
          }
          frame "----OPERATE----" {
          }
          frame "ready" {
          }
          frame "rx.start" {
            n128 = Variant To Data(type=T8 {"Samples"=0} ("RX.read config"), Variant=w271) -> (data=w269:T8)  [unwired: 1 in, 1 out]
            n129 = Unbundle By Name(w269) -> ("Samples"=w260:u32)
            "Samples" <- w260
            n130 = call "Read - Start.vi"("session in"=w261, "number of samples"=w260) -> ("session out"=w259:T22[], "error out"=w258:errorcluster)  [unwired: 12 in]
            n131 = Enqueue Element(queue=w268, element=T12 {"message"="ready", "data"=variant}, error in (no error)=w258) -> (error out=w263:errorcluster)  [unwired: 1 in, 2 out]
            n132 = Unbundle By Name(w263) -> ("status"=w266:bool)
            n133 = Select(t=HW_state_enum."configuration" ("hw state"), s=w266, f=HW_state_enum."running" ("hw state")) -> (s? t:f=w262:T13)
          }
          frame "exit" {
            n134 = call "Close.vi"("session"=w274) -> ("error out"=w273:errorcluster)  [unwired: 14 in]
            n135 = call <vilib>:"Clear Errors.vi"("error in (no error)"=w273) -> ()  [unwired: 5 in, 2 out]
          }
        }
        n136 = local write "State"(w184) -> ()
      }
      frame "running" {
        # "ACQUISITION STATE - each 1ms check for data and fetch it. remain ins tate until rx.stop command is recieved"
        n137 = Dequeue Element(queue=w287, timeout in ms (-1)=1) -> (element=w288:T12)  [unwired: 1 in, 3 out]
        n138 = Unbundle By Name(w288) -> ("message"=w284:string, "data"=w283:variant)
        n139 = case shown="Default" w284 {
          tunnel: w285 -> [w299 _ w325]
          tunnel: w283 -> [_ _ _]
          tunnel: [w299 HW_state_enum."configuration" ("hw state") w325] -> w282
          tunnel: w281 -> [w296 w320 w323]
          tunnel: [w298 w320 w323] -> w280
          tunnel: [w297 _ _] -> w279
          tunnel: ["running" ("State") "configuration" ("State") "closed" ("State")] -> w278
          tunnel: w277 -> [w289 _ _]
          tunnel: [_ _ TRUE] -> w276
          frame Default {
            # "no command recieved - check if data is available and fetch it"
            n140 = local read "Samples"() -> (w295:u32)
            n141 = call "Read - Check for available data.vi"("session in"=w296, "number of samples"=w295) -> ("session out"=w292:T22[], "data available"=w294:bool, "Elements Remaining"=→"Elements Remaining":u32, "error out"=w291:errorcluster)  [unwired: 10 in]
            n142 = case shown="True" w294 {
              tunnel: [w301 w311] -> w298
              tunnel: [w300 w302] -> w297
              tunnel: w295 -> [_ w309]
              tunnel: w292 -> [w301 w307]
              tunnel: w291 -> [w300 w306]
              tunnel: w289 -> [_ w304]
              frame False {
              }
              frame True {
                # "Send IQ data to SysA"
                # "read data\nfrom DMA"
                n143 = call "Read - Fetch IQ Data.vi"("session in"=w307, "number of samples"=w309, "error in"=w306, "Timeout (ms)"=500) -> ("session out"=w311:T22[], "data [channel]"=w310:cluster{"data":csg[]}[], "error out"=w303:errorcluster)  [unwired: 9 in]
                n144 = Index Array(array=w310) -> (element=w315:cluster{"data":csg[]})  [unwired: 1 in]
                n145 = Unbundle(w315) -> ("data"=w305:csg[])
                n146 = call-dynamic "SendData.vi"("error in (no error)"=w303, "data"=w305, "reference in"=w304) -> ("error out"=w302:errorcluster)  [unwired: 6 in, 2 out]
                n147 = Complex To Re/Im(x + iy=w305) -> (x=w314:sgl[], y=w313:sgl[])
                n148 = Build Array(w314, w313) -> (w316:sgl[][])
                n149 = case shown="True" "Plot" {
                  tunnel: w316 -> [_ w317]
                  frame False {
                  }
                  frame True {
                    "Waveform plot" <- w317
                  }
                }
              }
            }
          }
          frame "rx.stop read" {
          }
          frame "exit" {
            n150 = call "Close.vi"("session"=w323) -> ("error out"=w324:errorcluster)  [unwired: 14 in]
            n151 = call <vilib>:"Clear Errors.vi"("error in (no error)"=w324) -> ()  [unwired: 5 in, 2 out]
          }
        }
        n152 = local write "State"(w278) -> ()
      }
      frame "exit" {
      }
    }
    "error out" <- w142
    n153 = call <vilib>:"Simple Error Handler.vi"("type of dialog (OK msg:1)"=w140, "error in (no error)"=w142) -> ()  [unwired: 3 in, 5 out]
  }
  n154 = disable-structure shown="Disabled" {
    frame Disabled {
      n155 = flat-sequence {
        frame #0 {
          # "8"
          # "7"
          n156 = call <instrlib>:"niSync Disconnect Trigger Terminals.vi"() -> ("error out"=w331:errorcluster, "instrument handle out"=w330:refnum<k15>)  [unwired: 10 in]
          n157 = call <instrlib>:"niSync Close.vi"("error in (no error)"=w331, "instrument handle"=w330) -> ("error out"=w329:errorcluster)  [unwired: 9 in]
          n158 = call <vilib>:"Clear Errors.vi"("error in (no error)"=w329) -> ()  [unwired: 5 in, 2 out]
        }
      }
    }
    frame Enabled {
    }
  }
